vi "FIR Filter.vi"(7 "FIR Low-pass filter":T2={"Clip IIR filter ramps, 1/Fc"=1.0, "Two-pass & flip"=TRUE, "FIR filter specifications"={"Topology"=enum."Off", "Type"=enum."Lowpass", "#Taps"=50, "Lower PB"=100.0, "Upper PB"=0.0, "Lower SB"=200.0, "Upper SB"=0.0}, "optional FIR filter\n specifications"={"PB Gain"=-3.0, "SB Gain"=-60.0, "Scale"=TRUE, "Window"=enum."Flat Top"}} {"optional FIR filter\n specifications"."SB Gain" format="%.2p"; "optional FIR filter\n specifications"."PB Gain" format="%.2p"; "FIR filter specifications"."Lower SB" format="%0.2p"; "FIR filter specifications"."Upper SB" format="%0.2p"; "FIR filter specifications"."Lower PB" format="%0.2p"; "FIR filter specifications"."Upper PB" format="%0.2p"; "Clip IIR filter ramps, 1/Fc" format="%#_6p"}, 8 "error in (no error)":errorcluster, 9 "Settings":string, 11 "signal(s) in":waveform(dbl)[](array[waveform])) -> (0 "error out":errorcluster, 1 "Settings out":string, 3 "signal(s) out":waveform(dbl)[](array[waveform]), 4 "filter information":T1 {"phase H(w)"."df" format="%.2p"; "phase H(w)"."f0" format="%.2p"; "phase H(w)"."Phase H(w)" format="%.2p"; "magnitude H(w)"."df" format="%.2p"; "magnitude H(w)"."f0" format="%.2p"; "magnitude H(w)"."Mag H(w)" format="%.2p"})   [LabVIEW 2015]
uses:
  <vilib>/measure/macond.llb/FIR Filter for N Chan.vi
  <vilib>/Waveform/WDTOps.llb/WDT Waveform Duration DBL.vi
  <vilib>/Waveform/WDTOps.llb/WDT Get Waveform Subset DBL.vi
  <vilib>/measure/NI_MAPro.lvlib
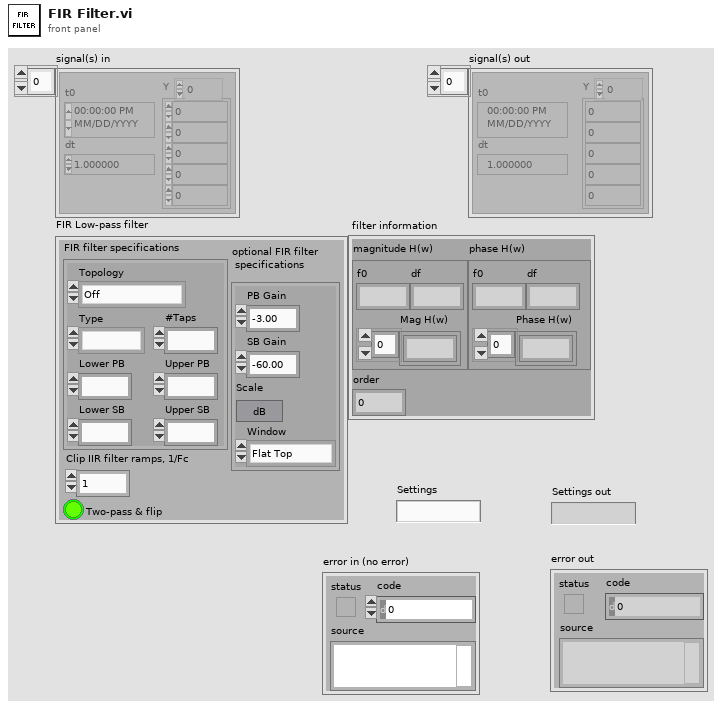
[diagram p1: front panel]
types:
  T1 = cluster{"magnitude H(w)":cluster{"f0":dbl, "df":dbl, "Mag H(w)":dbl[]}, "phase H(w)":cluster{"f0":dbl, "df":dbl, "Phase H(w)":dbl[]}, "order":i32}
  T2 = cluster{"Clip IIR filter ramps, 1/Fc":dbl, "Two-pass & flip":bool, "FIR filter specifications":cluster{"Topology":enum16{"Off", "FIR by Specification", "Equi-ripple FIR", "Windowed FIR"}, "Type":enum16{"Lowpass", "Highpass", "Bandpass", "Bandstop"}, "#Taps":i32, "Lower PB":dbl, "Upper PB":dbl, "Lower SB":dbl, "Upper SB":dbl}, "optional FIR filter\n specifications":cluster{"PB Gain":dbl, "SB Gain":dbl, "Scale":bool, "Window":enum16{"None", "Hanning", "Hamming", "Triangular", "Blackman", "Exact Blackman", "Blackman-Harris", "Kaiser-Bessel", "Flat Top"}}}
  T3 = cluster{"Topology":enum16{"Off", "FIR by Specification", "Equi-ripple FIR", "Windowed FIR"}, "Type":enum16{"Lowpass", "Highpass", "Bandpass", "Bandstop"}, "#Taps":i32, "Lower PB":dbl, "Upper PB":dbl, "Lower SB":dbl, "Upper SB":dbl}
  T4 = cluster{"PB Gain":dbl, "SB Gain":dbl, "Scale":bool, "Window":enum16{"None", "Hanning", "Hamming", "Triangular", "Blackman", "Exact Blackman", "Blackman-Harris", "Kaiser-Bessel", "Flat Top"}}
  T5 = enum16{"Off", "FIR by Specification", "Equi-ripple FIR", "Windowed FIR"}
  T6 = enum16{"None", "Hanning", "Hamming", "Triangular", "Blackman", "Exact Blackman", "Blackman-Harris", "Kaiser-Bessel", "Flat Top"}
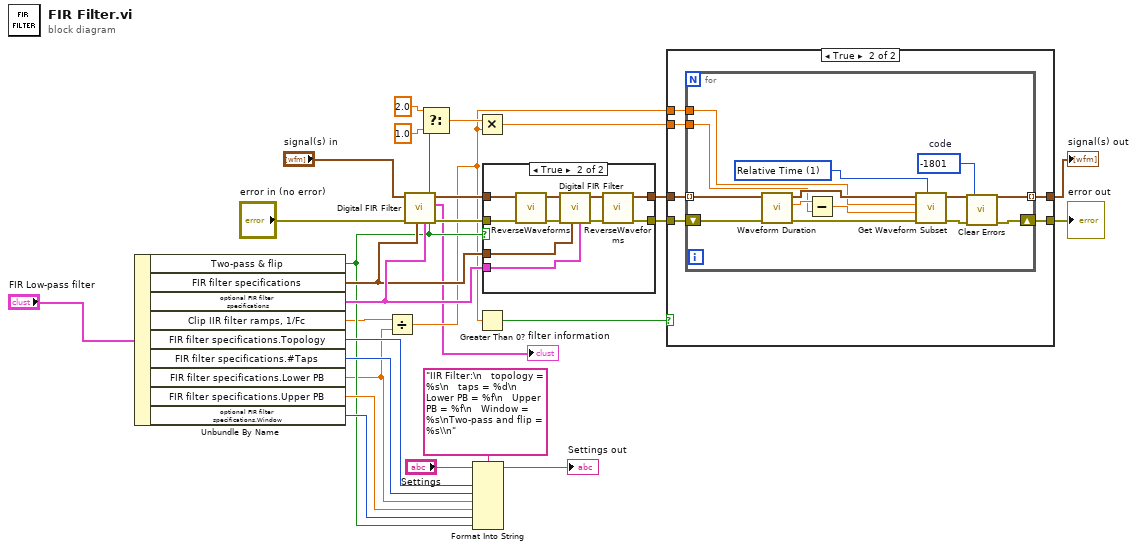
[diagram p0: block diagram]
diagram:
  n1 = Unbundle By Name("FIR Low-pass filter") -> ("Two-pass & flip"=w5:bool, "FIR filter specifications"=w13:T3, "optional FIR filter\n specifications"=w14:T4, "Clip IIR filter ramps, 1/Fc"=w3:dbl, "FIR filter specifications.Topology"=w9:T5, "FIR filter specifications.#Taps"=w8:i32, "FIR filter specifications.Lower PB"=w4:dbl, "FIR filter specifications.Upper PB"=w7:dbl, "optional FIR filter\n specifications.Window"=w6:T6)
  n2 = Divide(x=w3, y=w4) -> (x/y=w2:dbl)
  n3 = call-poly <vilib>:"Digital FIR Filter.vi"("optional FIR filter specifications"=w14, "FIR filter specifications"=w13, "error in (no error)"="error in (no error)", "signal(s) in"="signal(s) in") -> ("error out"=w27:errorcluster, "filter information"=→"filter information":T1, "signal(s) out"=w28:waveform(dbl)[])  [unwired: 5 in]
  n4 = Select(t=2.0, s=w5, f=1.0) -> (s? t:f=w19:dbl)
  n5 = Format Into String(format string="IIR Filter:\n   topology = %s\n   taps = %d\n   Lower PB = %f\n   Upper PB = %f\n   Window = %s\nTwo-pass and flip = %s\\n", initial string="Settings", w9, w8, w4, w7, w6, w5) -> (resulting string=→"Settings out":string)  [unwired: 1 in, 1 out]
  n6 = Multiply(x=w19, y=w2) -> (x*y=w18:dbl)
  n7 = Greater Than 0?(x=w2) -> (x > 0?=w17:bool)
  n8 = case shown="True" w5 {
    tunnel: w28 -> [w29 w38]
    tunnel: w27 -> [w30 w37]
    tunnel: [w30 w36] -> w23
    tunnel: [w29 w33] -> w24
    tunnel: w14 -> [_ w32]
    tunnel: w13 -> [_ w31]
    frame False {
    }
    frame True {
      n9 = call "ReverseWaveforms.vi"("signals in"=w38) -> ("signals out"=w34:waveform(dbl)[])  [unwired: 10 out]
      n10 = call-poly <vilib>:"Digital FIR Filter.vi"("optional FIR filter specifications"=w32, "FIR filter specifications"=w31, "error in (no error)"=w37, "signal(s) in"=w34) -> ("error out"=w36:errorcluster, "signal(s) out"=w35:waveform(dbl)[])  [unwired: 5 in, 1 out]
      n11 = call "ReverseWaveforms.vi"("signals in"=w35) -> ("signals out"=w33:waveform(dbl)[])  [unwired: 10 out]
    }
  }
  n12 = case shown="True" w17 {
    tunnel: w24 -> [w40 w46]
    tunnel: w23 -> [w39 w45]
    tunnel: [w40 w44] -> w22
    tunnel: w2 -> [_ w43]
    tunnel: w18 -> [_ w42]
    tunnel: [w39 w41] -> w15
    frame False {
    }
    frame True {
      n13 = for {
        tunnel: w46 -> [w55] mode=indexing
        shift-right: [w48] -> w41
        shift-left: w45 -> [w59]
        tunnel: [w58] -> w44 mode=indexing
        tunnel: w43 -> [w53]
        tunnel: w42 -> [w51]
        w47 = -1801  # code
        w56 = u16 1 items=["Samples", "Relative Time"] ("start/duration format")
        n14 = call-poly <vilib>:"Waveform Duration.vi"("error in (no error)"=w59, "waveform in"=w55) -> ("error out"=w57:errorcluster, "duration"=w52:dbl, "waveform out"=w54:waveform(dbl))  [unwired: 7 out]
        n15 = Subtract(x=w52, y=w51) -> (x-y=w50:dbl)
        n16 = call-poly <vilib>:"Get Waveform Subset.vi"("start/duration format"=w56, "error in (no error)"=w57, "duration"=w50, "start samples/time"=w53, "waveform in"=w54) -> ("error out"=w49:errorcluster, "waveform out"=w58:waveform(dbl))  [unwired: 3 out]
        n17 = call <vilib>:"Clear Errors.vi"("error in (no error)"=w49, "specific error code to clear (0: all)"=w47) -> ("error out"=w48:errorcluster)  [unwired: 4 in, 1 out]
      }
    }
  }
  "signal(s) out" <- w22
  "error out" <- w15
